vi "Read INI Cluster.vi"(8 "error in (no error)":errorcluster, 10 "INI Fomatted Cluster Type":variant, 11 "refnum":T1) -> (0 "error out":errorcluster, 1 "all found?":bool, 2 "INI Fomatted Cluster":variant, 3 "dup refnum":T1, 4 "any found?":bool)   [LabVIEW 2017, in "INI++.lvlib"]
doc: "Reads a cluster of section formatted clusters from configuration data identified by refnum, and returns them as a cluster of clusters of items. Section cluster names are used as section names and key-value pairs correspond to the named cluster elements and thier values within the section formatted clusters. Only the section clusters and items within the \"INI Formatted Cluster Type\" input cluster are read from the configuration data and returned in the output cluster of clusters of items. The \"found?\" output will be TRUE only if all elements (recursively) are found.\n\nFor example an Cluster containins subClusters MyCluster1 and MyCluster2, where MyCluster1 contains two elements MyNumeric and MyBoolean, and MyCluster2 contains two elements MyEnum and MyString. This would correspond to an INI write of the following data:\n\n[MyCluster1]\nMyNumeric=1.024\nMyBoolean=TRUE\n[MyCluster2]\nMyEnum=init\nMyString=\"Hello World\"\n\nNote: Special characters in section and key names will be escape-coded. These include the following: \\00-\\1F (non-printable chars); \"[\", \"]\", and \"=\" (INI syntax elements); \\FE (\"þ\") and \\FF (\"ÿ\") (legacy bracket encoding); Additionally, the escape character, \"\\\", will be escaped as \"\\\\\".\n\nNote: This VI checks whether every element of the cluster has a name so it can be identified."
uses:
  INI++.lvlib
  _openG/_reuse_openG.lvlib
  <vilib>/Utility/config.llb/Config Data RefNum.ctl
  <vilib>/Utility/config.llb/NI_LVConfig.lvlib
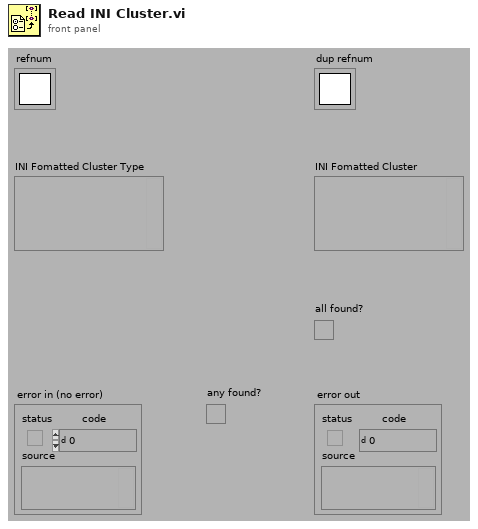
[diagram p1: front panel]
types:
  T1 = typedef "NI_LVConfig.lvlib/Config Data RefNum.ctl" = refnum<k1>
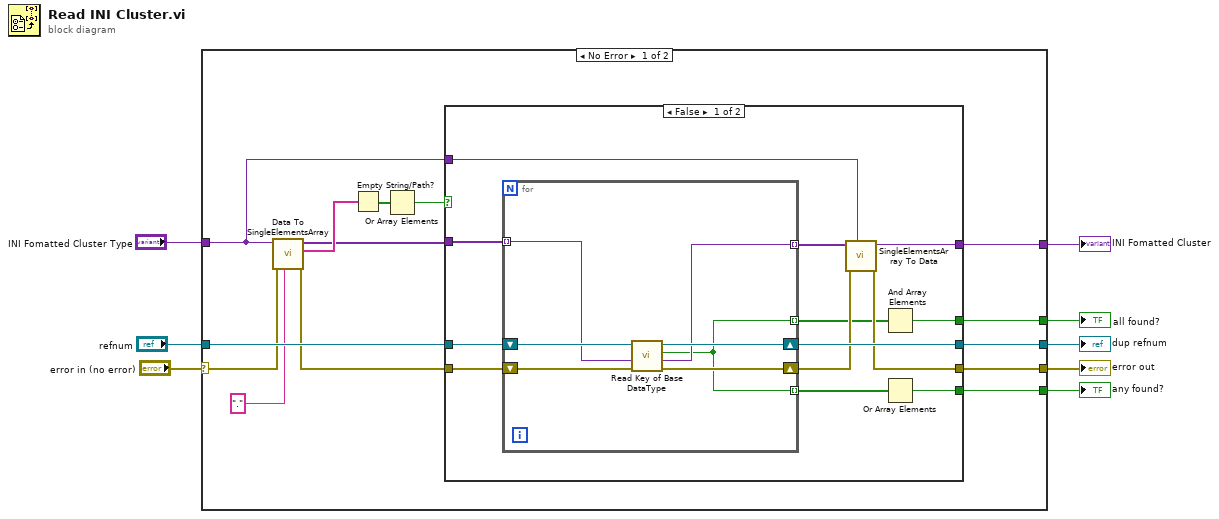
[diagram p0: block diagram]
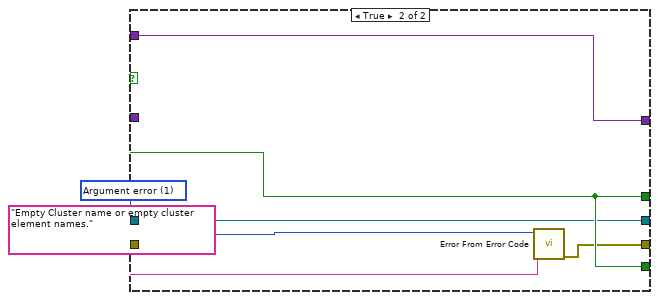
[diagram p2: hidden frame]
diagram:
  n1 = case shown="No Error" "error in (no error)" {
    selector: "error in (no error)" -> [w19 w51]
    tunnel: [w22 w50] -> w8
    tunnel: "refnum" -> [w21 w50]
    tunnel: [w20 w49] -> w6
    tunnel: "INI Fomatted Cluster Type" -> [w9 w49]
    tunnel: [w18 w51] -> w3
    tunnel: [w17 _] -> w2
    tunnel: [w16 _] -> w1
    frame No Error {
      n2 = call "Data To SingleElementsArray.vi"("Seperator(/)"=".", "error in (no error)"=w19, "Cluster"=w9) -> ("error out"=w10:errorcluster, "Full NameList"=w12:string[], "DataElementArray"=w11:variant[])  [unwired: 5 in, 1 out]
      n3 = Empty String/Path?(string/path=w12) -> (empty?=w15:bool[])
      n4 = Or Array Elements(Boolean array=w15) -> (logical OR=w14:bool)
      n5 = case shown="False" w14 {
        tunnel: [w35 w47] -> w22
        tunnel: w21 -> [w34 w47]
        tunnel: [w32 w43] -> w20
        tunnel: [w30 w44] -> w18
        tunnel: [w29 w48] -> w17
        tunnel: [w28 w48] -> w16
        tunnel: w11 -> [w25 _]
        tunnel: w10 -> [w24 _]
        tunnel: w9 -> [w23 w43]
        frame False {
          n6 = for {
            tunnel: w25 -> [w37] mode=indexing
            shift-right: [w39] -> w35
            shift-left: w34 -> [w42]
            shift-right: [w40] -> w31
            shift-left: w24 -> [w41]
            tunnel: [w38] -> w33 mode=indexing
            tunnel: [w36] -> w26 mode=indexing
            tunnel: [w36] -> w27 mode=indexing
            n7 = call "Read Key of Base DataType.vi"("error in (no error)"=w41, "type"=w37, "refnum"=w42) -> ("error out"=w40:errorcluster, "key-value"=w38:variant, "found?"=w36:bool, "refnum out"=w39:T1)  [unwired: 5 in]
          }
          n8 = call "SingleElementsArray To Data.vi"("Pototype"=w23, "error in (no error)"=w31, "DataElementArray"=w33) -> ("error out"=w30:errorcluster, "Cluster"=w32:variant)  [unwired: 7 in]
          n9 = And Array Elements(Boolean array=w26) -> (logical AND=w29:bool)
          n10 = Or Array Elements(Boolean array=w27) -> (logical OR=w28:bool)
        }
        frame True {
          w46 = 1 items=["No error", "Argument error", "Memory is full", "Out of zone", "End of file", "File already open", "Generic file I/O error", "File not found", "File permission error", "Disk is full", "Duplicate path", "Too many files open", "System feature not enabled", "Resource file not found", "Cannot add resource", "Resource not found", "Image not found", "Image memory error", "Pen does not exist", "Config type invalid", "Config token not found", "Config parse error", "Config memory error", "Bad external code format", "Bad external code offset", "External code not present", "Null window", "Destroy window error", "Null menu", "Print aborted", "Bad print record", "Print driver error", "Windows error during printing", "Memory error during printing", "Print dialog error", "Generic print error", "Invalid device refnum", "Device not found", "Device parameter error", "Device unit error", "Cannot open device", "Device call aborted", "Generic error", "Cancelled by user", "Object ID too low", "Object ID too high", "Object not in heap", "Unknown heap", "Unknown object (invalid DefProc)", "Unknown object (DefProc not in table)", "Message out of range", "Invalid (null) method", "Unknown message", "Manager call not supported", "Bad address", "Network operation in progress", "Network operation timed out", "Connection is busy", "Network attribute not supported", "Network error", "Address in use", "System out of memory", "Connection aborted", "Connection refused", "Not connected", "Already connected", "Connection closed", "Initialization error (interapplication manager)", "Bad occurrence", "Wait on unbound occurrence handler", "Occurrence queue overflow", "Datalog type conflict", "Unused", "Unrecognized type (interapplication manager)", "Memory corrupt", "Failed to make temporary DLL", "Old CIN version", "Drag socket not found", "Failed to load drop-object", "Failed to register OLE object", "Failed to release OLE object", "Format specifier type mismatch", "Unknown format specifier", "Too few format specifiers", "Too many format specifiers", "Scan failed", "Newer CIN version", "Error converting to variant", "Runtime menu error", "Password tampered", "Variant attribute not found", "Incompatible variant data type", "Event data is not available", "Event Store is not present", "Occurrence is not found", "Event Queue is not created", "Event info is not available", "Refnum passed is NULL", "Error retrieving Class GUID", "Error retrieving CoClass GUID", "Error retrieving TypeLib GUID.", "Bad built application magic bytes.", "Specific driver is different from the specific driver associated with the Logical Name.", "There is no session opened to the class driver.", "Max Error", "MAX - Error with config objects", "MAX - Error loading configuration", "MAX - Group not supported"]
          w48 = FALSE
          n11 = call "Error From Error Code.vi"("error message (\"\")"="Empty Cluster name or empty cluster element names." ("String to Prepend to source (\"\")"), "error code (0)"=w46) -> ("error out"=w44:errorcluster)  [unwired: 7 in]
        }
      }
    }
    frame Error {
    }
  }
  "error out" <- w3
  "dup refnum" <- w8
  "INI Fomatted Cluster" <- w6
  "all found?" <- w2
  "any found?" <- w1
